vi "Intake.vi"(6 "intake reversed?":bool, 8 "error in (no error)":errorcluster, 9 "Intake Running?":bool, 10 "Intake Out?":bool, 11 "Power Cell Handler in":refnum<class "Power Cell Handler.lvclass">) -> (0 "error out":errorcluster, 2 "Deploy Intake":bool, 3 "Power Cell Handler out":refnum<class "Power Cell Handler.lvclass">)   [LabVIEW 2019, in "Power Cell Handler.lvlib" / "Power Cell Handler.lvclass"]
uses:
  Power Cell Handler.lvclass
  <vilib>/Rock Robotics/WPI/ThirdParty/Phoenix-LabVIEW/Motor Controller/Controls/CTRE_Phoenix_MotorControl_ControlMode.ctl
  Power Cell Handler.lvclass/Power Cell Handler.ctl
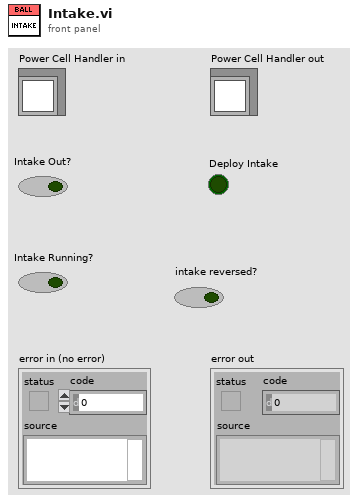
[diagram p1: front panel]
types:
  T1 = typedef "CTRE_Phoenix_MotorControl_ControlMode.ctl" = u16
  T2 = typedef "WPI_MotorControlDeviceRef.ctl" = cluster{"DeviceStatus":errorcluster, "Type":T3, "PWM":cluster{"PWM Channel":T4, "DeadBand":T5}, "CAN":cluster{"Device Number":u8, "SetOutput VI Ref":variant, "GetOutput VI Ref":variant, "Enable VI Ref":variant, "Disable VI Ref":variant, "Data":variant}, "Invert":bool, "DIO PWM":cluster{"PWM \"Enable\" Channel":T4, "DIOChannel":T6, "PWM Rate":dbl}}
  T3 = typedef "WPI_MotorControlType.ctl" = enum16{"PWM", "CAN", "DIO PWM"}
  T4 = typedef "FPGA_DIOPWMChannel.ctl" = enum8{"PWM 0", "PWM 1", "PWM 2", "PWM 3", "PWM 4", "PWM 5", "PWM 6", "PWM 7", "PWM 8", "PWM 9", "PWM MXP 0", "PWM MXP 1", "PWM MXP 2", "PWM MXP 3", "PWM MXP 4", "PWM MXP 5", "PWM MXP 6", "PWM MXP 7", "PWM MXP 8", "PWM MXP 9", "Invalid"}
  T5 = typedef "WPI_PWMDeadband.ctl" = cluster{"Name":string, "maxPositivePwm":i32, "minPositivePwm":i32, "centerPwm":i32, "maxNegativePwm":i32, "minNegativePwm":i32, "angularRange":u16}
  T6 = typedef "FPGA_DIOChannel.ctl" = enum8{"DIO 0", "DIO 1", "DIO 2", "DIO 3", "DIO 4", "DIO 5", "DIO 6", "DIO 7", "DIO 8", "DIO 9", "DIO MXP 0", "DIO MXP 1", "DIO MXP 2", "DIO MXP 3", "DIO MXP 4", "DIO MXP 5", "DIO MXP 6", "DIO MXP 7", "DIO MXP 8", "DIO MXP 9", "DIO MXP 10", "DIO MXP 11", "DIO MXP 12", "DIO MXP 13", "DIO MXP 14", "DIO MXP 15", "SPI Port CS1", "SPI Port CS2", "SPI Port CS3", "SPI Port MISO", "SPI Port MOSI", "Invalid"}
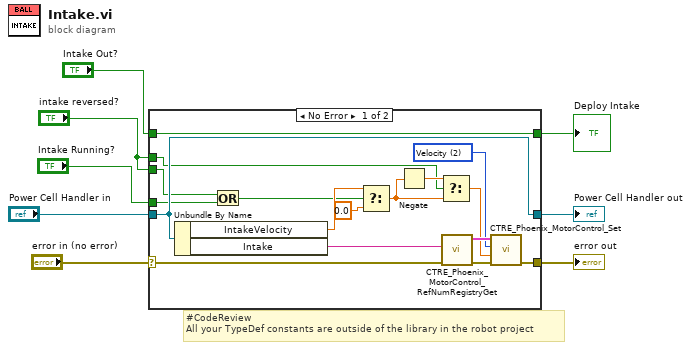
[diagram p0: block diagram]
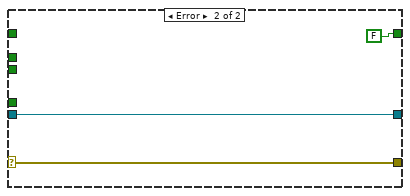
[diagram p2: hidden frame]
diagram:
  # "#CodeReview\nAll your TypeDef constants are outside of the library in the robot project"
  n1 = case shown="No Error" "error in (no error)" {
    selector: "error in (no error)" -> [w18 w28]
    tunnel: [w17 w28] -> w7
    tunnel: [w25 w27] -> w5
    tunnel: "Power Cell Handler in" -> [w25 w27]
    tunnel: "Intake Running?" -> [w16 _]
    tunnel: "Intake Out?" -> [w15 _]
    tunnel: [w15 FALSE ("Intake Out?")] -> w1
    tunnel: "intake reversed?" -> [w13 _]
    tunnel: "intake reversed?" -> [w10 _]
    frame No Error {
      w21 = T1 2 items=["PercentOutput"=0, "Position"=1, "Velocity"=2, "Current"=3, "Follower"=5, "MotionProfile"=6, "MotionMagic"=7, "MotionProfileArc"=10, "Disabled"=15] ("Control Mode")
      n2 = Unbundle By Name(w25) -> ("IntakeVelocity"=w19:dbl, "Intake"=w24:string)
      n3 = Or(x=w13, y=w16) -> (x .or. y?=w14:bool)
      n4 = Select(t=w19, s=w14, f=0.0) -> (s? t:f=w9:dbl)
      n5 = Negate(x=w9) -> (-x=w11:dbl)
      n6 = Select(t=w11, s=w10, f=w9) -> (s? t:f=w12:dbl)
      n7 = call <vilib>:"CTRE_Phoenix_MotorControl_RefNumRegistryGet.vi"("error in (no error)"=w18, "refnum name"=w24) -> ("error out"=w23:errorcluster, "PhoenixMotorControlDevRef"=w22:T2)  [unwired: 8 in]
      n8 = call <vilib>:"CTRE_Phoenix_MotorControl_Set.vi"("error in (no error)"=w23, "Output"=w12, "Control Mode"=w21, "PhoenixMotorControlDevRef"=w22) -> ("error out"=w17:errorcluster)  [unwired: 6 in, 1 out]
    }
    frame Error {
    }
  }
  "error out" <- w7
  "Power Cell Handler out" <- w5
  "Deploy Intake" <- w1
